vi "MGI Fade In & Out.vi"(7 "Error In":errorcluster, 8 "Speed (3)":dbl=3.0, 9 "Fade (In)":enum16{"In", "Out"}(ring), 10 "VI Reference In (Top Level)":refnum<vi>) -> (0 "Error Out":errorcluster, 3 "VI Reference Out":refnum<vi>)   [LabVIEW 2016]
doc: "This VI iteratively sets the transparency of the referenced VI from fully transparent to fully opaque and vice versa, providing a visual \"Fade In\" or \"Fade Out\". The default \"Speed\" is set at an arbitrary '3'. A higher number will cause a faster fade.\n\nAuthored by Robert C. Mortensen\nsupport@mooregoodideas.com\nwww.mooregoodideas.com\n\nCopyright (c) 2010, Moore Good Ideas, Inc.\n\nAll rights reserved.\n\nRedistribution and use in source and binary forms, with or without modification, are permitted provided that the following conditions are met:\n\n * Redistributions of source code must retain the above copyright notice, this list of conditions and the following disclaimer.\n * Redistributions in binary form must reproduce the above copyright notice, this list of conditions and the following disclaimer in the documentation and/or other materials provided with the distribution.\n * Neither the name of Moore Good Ideas, Inc. nor the names of its contributors may be used to endorse or promote products derived from this software without specific prior written permission.\n\nTHIS SOFTWARE IS PROVIDED BY THE COPYRIGHT HOLDERS AND CONTRIBUTORS \"AS IS\" AND ANY EXPRESS OR IMPLIED WARRANTIES, INCLUDING, BUT NOT LIMITED TO, THE IMPLIED WARRANTIES OF MERCHANTABILITY AND FITNESS FOR A PARTICULAR PURPOSE ARE DISCLAIMED. IN NO EVENT SHALL THE COPYRIGHT OWNER OR CONTRIBUTORS BE LIABLE FOR ANY DIRECT, INDIRECT, INCIDENTAL, SPECIAL, EXEMPLARY, OR CONSEQUENTIAL DAMAGES (INCLUDING, BUT NOT LIMITED TO, PROCUREMENT OF SUBSTITUTE GOODS OR SERVICES; LOSS OF USE, DATA, OR PROFITS; OR BUSINESS INTERRUPTION) HOWEVER CAUSED AND ON ANY THEORY OF LIABILITY, WHETHER IN CONTRACT, STRICT LIABILITY, OR TORT (INCLUDING NEGLIGENCE OR OTHERWISE) ARISING IN ANY WAY OUT OF THE USE OF THIS SOFTWARE, EVEN IF ADVISED OF THE POSSIBILITY OF SUCH DAMAGE."
uses:
  <userlib>/_MGI/Application Control/MGI VI Reference/MGI Caller's VI Reference.vi
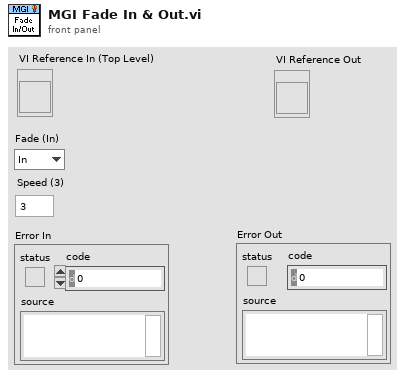
[diagram p1: front panel]
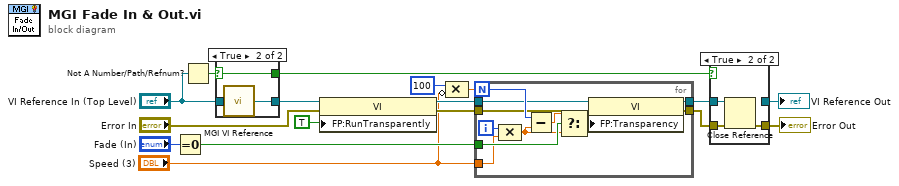
[diagram p0: block diagram]
diagram:
  n1 = Equal To 0?(x="Fade (In)") -> (x = 0?=w10:bool)
  n2 = Not A Number/Path/Refnum?(number/path/refnum="VI Reference In (Top Level)") -> (NaN/Path/Refnum?=w3:bool)
  n3 = case shown="True" w3 {
    selector: w3 -> [_ w19]
    tunnel: [w18 w20] -> w5
    tunnel: "VI Reference In (Top Level)" -> [w18 _]
    tunnel: [_ w19] -> w2
    frame False {
    }
    frame True {
      n4 = call-poly <userlib>:"MGI VI Reference.vi"() -> ("Caller's VI Reference"=w20:refnum<vi>)  [unwired: 1 in]
    }
  }
  n5 = property class="VI"(reference=w5, error in="Error In", "FP:RunTransparently"=TRUE ("Front Panel Window:Run VI Transparently")) -> (reference out=w15:refnum<vi>, error out=w14:errorcluster)
  n6 = Compound Arithmetic op=MULTIPLY(100, invert "Speed (3)") -> (w8:dbl)
  n7 = for {
    N: w8 -> [w30]
    tunnel: [w31] -> w12
    tunnel: [w29] -> w13
    tunnel: w15 -> [w28]
    tunnel: w14 -> [w27]
    tunnel: w10 -> [w26]
    tunnel: "Speed (3)" -> [w21]
    i -> [w23]
    n8 = Compound Arithmetic op=MULTIPLY(w23, w21) -> (w22:dbl)
    n9 = Subtract(x=w30, y=w22) -> (x-y=w24:dbl)
    n10 = Select(t=w24, s=w26, f=w22) -> (s? t:f=w25:dbl)
    n11 = property class="VI"(reference=w28, error in=w27, "FP:Transparency"=w25) -> (reference out=w29:refnum<vi>, error out=w31:errorcluster)
  }
  n12 = case shown="True" w2 {
    tunnel: [w33 w36] -> w17
    tunnel: w13 -> [w32 w35]
    tunnel: w12 -> [w33 w34]
    tunnel: [w32 _] -> w1
    frame False {
    }
    frame True {
      n13 = Close Reference(reference=w35, error in (no error)=w34) -> (error out=w36:errorcluster)
    }
  }
  "Error Out" <- w17
  "VI Reference Out" <- w1
